vi "Main_04A.vi"() -> ()   [LabVIEW 2025]
uses:
  Utility/Universal Utility/TypeDefs_Utility/ENUM_8 Directions U-D-L-R.ctl
  Utility/Universal Utility/TypeDefs_Utility/Cluster_Row-Column.ctl
  b43e3300-6143-4e08-a70a-80936fe279ff.vi
  9e3f57c0-2ef8-4495-8287-c6a42a5fb955.vi
  <vilib>/Utility/error.llb/Trim Whitespace.vi
  <vilib>/Utility/error.llb/Trim Whitespace One-Sided.vi
  Utility/Universal Utility/TypeDefs_Utility/ENUM_4 Directions U-D-L-R.ctl
panel:
  out "Array":bool[][](array[boolean])
  out "MATCH":bool
  in  "Select Data":enum32{"Example", "Puzzle"}(tab)
  in  "EX Target":u32=13
  in  "Example":string="..@@.@@@@.\n@@@.@.@.@@\n@@@@@.@.@@\n@.@@@@..@.\n@@.@@@@.@@\n.@@@@@@@.@\n.@.@.@.@@@\n@.@@@.@@@@\n.@@@@@@@@.\n@.@.@@@.@."
  in  "Puzzle":string="@@..@.@.@..@@.@@@@@.@@@@@@..@@.@@.@@..@@@.@@@.@.@@@@.@@@.@@@.@..@.@@@@..@@@.@@..@@@.@@@..@@@@..@.@@.@@@.@..@.@@@.@@@..@@@.@.@@@@@.@.@.@@@@@@\n@.@@@@@@....@..@@@.@..@.@.@@.@@.@@..@@@..@.@@..@..@@@.@@@.@..@.@.@@..@@.@..@@.@@@..@.@@.@.@..@@...@@@@@@@@.@@@.@@@.@@.@@@@@@@..@..@@@.@.@@.@\n.@.@@@@.@@.@@.@.@.@@.@..@@.@@..@@@@@@@@@@@@...@@.@...@@@@.@.@@.@@@.@.@@..@@.@@.@@.@@..@...@@@@.@@@@@@@@@@@.@@@....@@@@@.@.@...@@.@@@@@@@.@@@\n@@@..@@@@.@@@@@@@@.@@@@@.@@.@....@.@..@.@@@@@@@...@@@@@@@@.@@...@.@@.@@@@@@.@....@@.@@@.@.@@..@@@.@.@@@..@.@.@@@.@.@@@@@@@@...@.@@@@@@.@..@@\n@.@@@@@.@@.@.@.@.@..@@@@.@..@...@.@@@.@.@@@@.@@.@@@@@@.@@@@@..@@..@.@.@@.@.....@@@.@@@.@..@@@.@@.@..@@@@.@.@@@@..@@@@@@.@@@.@@.@@..@@.@.@@@@\n@@.@@@@@.@@@.@@@@@.@@.@.@@@@.@@...@.@@@..@@.@@.@@@..@@@...@@.@@@@..@@@@@@@...@.@@@@@@....@..@@@@@.@...@.@.@@.@...@@@@.@.@@@.@@.@.@@@@.@.@@@@\n...@.@@.@@.@.@.@@@@...@@@@@@@@@.@.@@@.@@.@@@.@@.@@@@.@@@@@@@@@.@@..@..@.@@@@@@@@@@@@...@.@.@@@.@.@.@.@@@.@..@@@@@@@@@@@.@@.@...@@@@@@@@.@@@@\n..@@@.@.@.@@@@@...@@..@@..@@.@...@@@.@.@.@.@.@@.@.@@@.@@.@.@@@@.@.@@@@@@@.@@.@.@@@@@@.@.@@@@@@@@@@@.@.@@@@@.@@@@@@@@@.@...@@@.@@@@.@..@@@@..\n.@@@@.@@@.@.@@@.@@@..@@..@@@@@@.@..@.@@.@.@@@@@..@@@@@@@@.@.@@@.@@@@@.@.@@@@...@@.@@@.@.@@@@@@.@@.@.@@@@.@.@@@.@.@@@@@.@@@@...@@@@@@@@@@.@..\n@.@....@@.@..@@@.@.@..@@@@.@.@@.@..@@.@.......@.@@@@@@@.@@@@@@@@.@@@.@.@@.@@@@.@..@.@@@@@@.@@@@....@@.@@@@.@..@@@.@@.@.@@@@@@@@.@@@@.@.@@..@\n@@@@@.@@.@.@.@@.@..@@@.@.@@@@.@@@.@.@.@@@.@.@@@.@@@@@..@@@@@@..@@@@@@@@@@@@@@.@@@@.@@@@...@.@@@@..@@@@@@@.@@@@.@@.@@@@@@.@@@.@.....@@@@@@.@.\n@.@@...@@@.@@..@@@@..@@.@@.@...@@@@@...@@@@.@@@.@@.@..@@@@..@.@@@@..@@@.@..@@@@..@.@@.@.@.@@....@.@@..@@.@@..@@@@...@@.@..@@@@@@@...@@@..@.@\n...@.@...@@@..@..@.@@@@.@.@....@@@@@@.@..@@@@@.@@@@@@@@@@.@@@@@@@@.@@..@@@@@@@@@@@@@@.@.@...@@....@@.@@.@@@.@@@@@@.@.@..@@@@@@.@.@.@@..@@@@.\n@@@@.@@@@.@.@@.@.@..@@@..@@@.@@@@@..@@@@@@.@...@.@@@.@.@..@@@@@@.@@.@@@.@@..@@@@@@@..@@@@@@@@..@@..@@@@@..@.@.@@@.@@..@.@.@@@@@@@.@.@@@.@@@.\n@@@@@@@@.@@@@@@@.@@@.@.@.@@.@..@@@@@@@.@@..@@..@.@..@.@@@@@@..@.@.@@.@.@@@.@.@@@@..@@@@@@@@....@.@.@@@@@@@@@.@@@..@@@@@@..@@@@...@@@...@.@.@\n..@@@..@.@@.@.@@...@@@..@.@@@...@..@@.@@@@@..@@@@.@@@@.@@@.@@.@@.@@@@@@@..@.@..@.@.@@@..@@@@@...@@..@....@......@.@.@.@.@@@.@.@@@@@@@.@@.@@.\n.@@.@@@@@.@..@@@@@@.@....@@@.......@..@@@.@@@...@..@@..@@@@..@.@@@@.@@.@@..@@.@.@@@@.@@.@@.@@@@@...@@@@.@@@..@.@.@@@.@.@@.@@@..@@@..@@@@@..@\n@.@.@..@.@.@.@@.@@@@@@@@@@@@.@@@@.@@..@.@.@@@..@@@@.@@@@@...@.@@.@@@@@@@...@@..@@@@..@@....@.@@@.@.@@@@@.@@@@@@@..@@@@@@@@@.@@@@..@@@.@....@\n@@..@@.@@.@.@..@@...@.@.@.@@....@@@@@@.@.@@@@@@.@..@@@@@@.@@@@..@.@.@.@.@.@@.@@...@@@.@.@@.@@.@@@@@@@.@..@@.@.@.@@..@.@@@@@@@@.@@@@..@@...@.\n.@@..@@@@@@@.@.@@@@.@@@@@@@@.@.@@@@@@@@@.@@@@@.@@@@..@@@@..@.@@@@.@.....@.@@.@@.@@@@@..@@@@@.@@@@@.@@@.@@.@@@..@@@..@@@@.@@.@@@@@@@@@@@@.@@@\n.@..@@@@@@@@@@@.@@.@@.@..@..@@@...@@..@@@.@@.@.@@.@.@..@@.@@.@@@@@.@@@.@.@@@@.@@@@@.@...@@.@@.@.@@..@@@.@@@@@.@@@@@.@....@@@@@@@@.@@.@@@@@@@\n@..@@..@@@@.@@.@.@.@.@.@@@@..@@.@..@.@@@@@@@.@@..@@@@@.@@@.@@@.@.@@.@@.@@@.@@@@@@@@@@@@@.@@@@@@.@@@@@@@...@@@@@@@.@@@@.@.@.@@@.@@@.@..@@@..@\n@@@@@@@@.@.@@..@.....@.@@@...@.@@..@@@..@..@..@@@.@@@@@@@@.....@..@@.@.@.@.@@@@.@@.@@.@@@@@@.@.@.@@.@@@@@.@.@@@...@@.@@@@@@@...@.@@.@@@..@.@\n.@@@@@@..@.@@...@@@@@@@@@@@.@@@@@..@...@.@.....@@@.@.@@@.@@...@.@.@.@@@@@@.@@@@@@.@@@@@...@@@@.@..@@.@@@.@@.@.@@@..@@@@@@@@.@@@.@@..@.@.@.@@\n@.@@.@@@.@.@.@.@@@@@@@@.@@@@..@.@@@@@.@@.@@....@..@@.@..@@@....@@..@@.@@@@@@@@@....@@.@@@.@@..@...@@@@@@@.@@@@@.@@@.@@@@@@@@@@...@@.@.@@@@@@\n@@@@@@@@@...@.@.@@@.@@.@@.@.@..@..@..@..@.@.@@@.@@@@@@@@@...@@@@@@@@@@.@@@.@@.@@...@@@@@@@.@.@@.@@@@@.@.@@..@..@....@.@@@.@...@..@..@@.@@@@@\n@@@@@@@@...@@@.@@@....@@@.@..@@@@.@@@@@..@@@...@@.@.@@@.@@.@.@@.@.@@@@.@@.@@@@@@@@@@@@..@@....@@.@@@@@.@@@@@....@@@....@@@@@.@.@@.@@..@@@@@@\n.@@@@.@@@@....@..@.@@@@@.@@@@@@..@..@@.@@@@.@@@..@@@...@.@@@.@.@@@@@@@..@..@...@@@.@@@.@@@..@@@@@...@...@..@@@@@.@@..@@...@@@.@@@@@.@@@...@@\n@..@@@...@@@.@.@@@@.@@@@@@.@@@@.@@.@@@@@@@..@@@..@@@@.@@@@..@@@..@.@@@...@@.@@@@..@@@@@@@@.@@@.@@...@@...@.@..@.@.@@.@.@@@@.@@.@..@@..@..@@.\n@@@@@@@..@@..@@.....@@..@@@..@@@@@..@@@@@.@@@@@.@..@@@@..@.@@@@...@..@@@.@.@@@..@@@..@@@@@..@@@@.@.@.@@.@@@@@@...@@@@@@@@@@..@@.@.@@.....@@@\n.@@@@......@@@.@@..@@@.@..@.@@@@@@.@.@..@@.@@@.@@@@....@@@@.@@.@@@@@@@.@.@@@..@@@.@@@@@@..@@@.@@@@.@@@@@.@@@@@@@.@@.@@@@@@.@@@@@@@@@.@..@@@@\n....@@@@@.@.@@@@@@@@@.......@.@@@@@@..@@.@@@@.@@@..@@@.@..@@@.@.@@.@@@.@@..@@@.@@@@@@@.@.@@@@@@...@@.@..@.@@.@.@@.@@@@@.@@@@@.@..@...@@@.@@@\n@@@@@@@@@@@@.@@.@@@.@@.@@.@@@..@@@@@.@@@.@..@.@.@@.@@.@@@@@..@@.@@..@....@..@...@@@@@..@..@.@.@@..@...@@@@..@.@@@@@@@@.@@@@@@@@@.@..@.@@@@@.\n@.@..@@@@..@@.@@.@.@@@@@..@@@@@@@....@@.@@..@@.@@@@...@@@@.@@@@@@@@@@.@.@@.@..@.@@@@@@@@.@@@..@@..@..@@@..@@@@....@@@@@@.@@..@@@@@@@@@@@@@@.\n.@@.@.@.@@@@@@.@@@.@@@@.@..@.@@.@@@@..@@@@@@.@@@.....@.@.@....@.@@@@@.@@@@.@@@@@@@@@@.@@@.@@@@@@@..@@..@@.@...@.@@@.@.@.@@.@.@@@@@@..@@@@.@@\n@.@@.@@@@@@@@@.@.@@.@@@@@@@.@@....@@.@@.@@@@@.@@@@.@...@@.@@@@.@@@@@.@..@@@@@@@.@@..@@@@@..@@.@...@@.@@.@@@@.@@@@..@..@@@@@.@@@.@@.@@@@@...@\n@.@@@.@.@..@.@@.@.....@.@.@@@@@@@@@.@@@@@@@@@@.@..@.@@.@@...@@@.@.@@.@.@.@@.@@@..@@@@@@.@@@@@@@@@.@....@.@@@@@@.@@@@@.@@.@.@@@@@@@.@@@@@@@.@\n@.@...@@@...@@.@@..@@..@.@.@@..@.@.@..@..@@@@@@@..@@@@@@@@@@.@@.@@@.@@@@..@..@.@@..@@@.@.@.@@@.@.@.@@@@@@....@.@@@@@@@@@.@@@@@@..@@@.@@@.@@@\n.@@@@.@@@.@.@.@@..@@@.@@@@..@@@.@@.@@@..@@@.@@..@.@@@@@@..@@@@@.@@@.@@..@.@.@@@@...@@.@...@.@@@.@@@@.@@@.@..@@@@..@@@..@@.@@.@.@@.@.@.@@.@@@\n..@@@@..@@@..@.@@@@@.@..@.@@.@...@@@@@@@@..@.@@@@@@...@@@@.@.@@@....@...@@.@..@@@@@.@.@.@.@@.@@@@@.@@@@@..@@@@@@@..@@.@@.@@..@...@@@@@@@.@.@\n.@@@@.@@@@.@@@@@..@..@@..@.@.@@....@@@@.@...@@@@@@@@..@.@..@.@@@@@@@@@@@.@.@@..@.@@.@.@@@@@@.@@@.@@@.@@@..@@..@@..@.@@...@@.@..@..@.@@@.@.@@\n.@@@@@@@@@@@@.@@@.@@...@..@..@..@.@.@@@.@..@.@@...@@.@@..@@@@@@..@@@@@@@.@.@@@@@.@@.@...@@.@@.@@@@@@.@@@.@.@@@@..@...@@@@...@@.@@@@@@@@.@@.@\n.@@@@.@..@..@.@@@@@.@.@@@@.@.@.@.@..@.@@@@..@@@..@@..@..@@@@@.@.@@@@...@..@....@..@@.@...@@.@.@@@.@@@@.@@@.@@@@@....@@@@.@@@.@..@@@@@@@..@.@\n@@@@@@@@.@@@...@@..@.@.@.@@.@@.@@..@@@..@@.@@@@@@.@@.@@...@.@@@@..@@@@@..@@..@.@@@@@@@@@..@@...@@.@@@.@@@@@@@.@@..@@.@@@@.@...@.@.@..@@.@.@@\n@.@@@.@.@@@@@@@@@@@..@@...@.@@@..@@@@@..@.@@@..@.@@@@.@@@@@@@@@.@.@@@.@@@@@@@..@.@@...@@@..@@.@.@@.....@@@.@@.@..@@.@..@@@.@.@.@.@@@.@@.@@@@\n@.@.@....@@@.@@..@@@.@@@@@@@.@.@@.@.@@@@@@@.@@.@@@@@.@.@@....@.@@@..@@@@@.@@@@.@.@@@.....@@@@@@@@@@..@..@@@@@@..@.@@@@@@@.@.@@.@@@.@@@@.@.@@\n.@@@@.@@@.@..@@@.@@@.@..@@.@@.@.@@.@@@.@.@@@@@.@@.@..@.@.@@@@.@@@.@@.@@@..@.@.@@@..@@@@@@@@@@@.@@@@@@@@@.@@@@@@..@@@...@@@.@@.@.@@@@@@.@@@@@\n@@.@.@@@@@@@@@..@@...@@@@..@@@.@@.@.@.@@....@@..@@.@@..@@@.@@.@..@@.@@@@.@@@@@@@@.@@@@@@@@@..@.....@@@@....@@@@@...@...@..@@@@@.@@.@....@.@@\n.@@.@@...@@@@@@.@@.@@@@.@.@@@@.@@.@..@@@@.@...@@@@.@.@....@.@@@@@@@@@.@@..@@.@.@@@@@@.@.@@.@.@@@@@@....@.@@@@@.@.@.@.@@@@..@@@@.@.@..@..@@@@\n.@@@@@.@@@.@.@@...@@..@@@..@@...@@@@..@...@.@...@@.@.@@@@...@@@..@@@@@@@@@.@@.@..@.@.@@.@@@.@@@..@@@@...@@@@@@@..@.@@@@@@.@@.@.@@@@.@...@@.@\n@@..@.@.@@.@.@@.@.@@@..@@...@@@@@@@@@@.@.@@@@@@.@.@.@@..@@@..@...@@@@..@......@.@.@..@.@.@.@.@@@@.....@.@.@.@@.@@.@.@@@@@@.@@@@@..@.@.@..@@@\n.@@@@@@@@@@.@@@@..@.@.@.@@@@@@@@.@@@.@@.@@..@@..@@@.@@..@.@.@.@@@..@.@.@@@.@..@@@.@@.@.@..@@@...@.@@@@...@@@.@.@@.....@@...@.@@.@@@@@.@@@@@.\n.@@@..@@@@@@@.@@@.@@@@..@@@..@..@@@..@@@..@@.@@.@@@@@@@.@.@@@.@.....@@@@@.@@.@@..@@@@.@@....@@@..@@@@.@@@@@@.@@.@..@@@.@..@@..@..@@.@@@.@@..\n@@@@@@..@.@@@@@.@@@@.@..@.@@@@@..@@@@..@..@@@@@.@@@@@@@.@..@@..@@@@@@@@..@@@@.@.@@.@@...@.......@@.@..@@@@.@..@@@@...@.@@@.@......@@...@@@..\n@.@.@.@....@.@.@@.@@@@@@@.@..@.@..@@.@.@.@@@@@@..@...@...@.@.@.@.@@@@@@@@@..@@@.@@@@@@@@@.@..@@@@@@.@@.@@@@@@.@@.@@...@@@@@@.@@@.@@.@..@..@@\n.@@@.@@@@@@@@.@@@.@..@@.@..@..@@.@@@..@@@@@@.@@@@..@@....@@@@.@.@@.@@.@@@..@@@@@@@....@..@@.@@@@@..@..@...@@.@@@@@.@@.@@@@.@@@@@@.@..@.@@@.@\n@..@...@@@@..@@..@@..@@@.@.@@@@.@..@@@.@.@.@@@@@.@@...@..@@...@....@.@.@@@@@.@@@.@@..@@.@@@.@.@@..@@@@..@@@@@@@@@.@@@@@.@@.@@.@.@@.@.@.@@@.@\n@.@.@@@.@..@.@.@.@.@@@@@@@.@.@@.@..@@@.@@@@@@@...@@@.@@@.@@@@.@@@....@@@@@@@.@@.@.@@...@..@@.@..@.@@.@.@@@@..@@@.@@@@@@..@@@..@.@@@@@@@@@@.@\n.@@.@@@@..@..@@.@.@.@@.@@@@..@@.@....@@@@.@@@.@@@.@@@@@@@@.@@.@@@.@@@@.@@@@@@@@@.@@@@..@@.@..@@@.@.@@@@@@@@@@@.@@.@.@.@...@@@@@.@@.@...@@@@@\n.@..@@...@@.@@@@@@@@@@.@@@.@@.@@@@@@@.@@.@@@@.@@..@@.@.@@.@@@.@@@@.@.@@@@..@...@.@...@@@.@@@@@..@@@@@@@..@.@@@.@.@.@.@.@@.@@@@..@.@..@.@.@@.\n.@..@...@.@@.@..@@@@@@..@.@@@@@@...@@..@@.@@@@.@....@.@@@..@@@@..@@.@.@..@.@@.@.@.@@@.@..@.@@@@@@.@@@.@@.@.@..@@.@@.@.@@@.@.@.@.@@@.@@@.@@..\n.@@@.@.@..@..@@@..@@@.@@.@.@@@.@@@.@@@.@@@..@@@@@@..@@@@@@@.@@@@.@.@...@@@@@@@.@@@@...@..@@@@.@.@@@......@@@.......@@.@..@@@@@..@.@.@@@...@@\n.@@@@@@.@@@.@@@@@@@.@@.@@.@@@@@..@.@.@.@..@@.@.@.@@@.@.@@@.@@@.@@.@@..@@@..@@@@...@@..@.@.@@@..@@..@.@@@.@..@.@@@@@@@@@...@@@@.@@@@@@@.@.@.@\n@.@.@@.@@@....@@@@@@@.@@@...@@@..@.@@@@@@@@@@@@.@.@@@@@.@@@.@@.....@.@@@....@.@@....@@@@@@@.@@@@@.@@@.@.@.@@.@@@@@@@@..@.@.....@@@@@..@@@@.@\n@....@...@.@.@..@@@@@......@.@...@.@.@..@@.@@@@@@..@@@@.@.@.@.@.@.@...@@@@.@@@.@...@...@@@...@@@@@@@@@@@..@@@..@.@@@@@@.@@@@@....@@@.@@.@..@\n@@@@.@..@@@.@@@..@@.@@@@@@.@.@.@.@@@@@@@.@.@@.@@@.@@...@@.@.@.@@..@@@.@@@@@.@@.@.@@@@@.@@@@@@.@@.@@@@@.@.@@.@@....@@....@....@@@@.@@.@@@..@@\n@.@@@@@@@@@..@@@@@..@.@@.@..@@@.@@@@@@@@..@@@@@..@@@.@.....@@@..@.@@@@@@..@@..@@@.@.@..@.@@.@@@@@@.@.@@.@@@.@@.@@.@..@.@.@@@@..@.@@@@..@.@.@\n@@@@@.@.@.@@...@@...@@@@@@@@.@..@..@@@@..@@@..@.@@.@.@@@.@.@@@...@.@@@..@@@@@@@@@....@@@@@.@@@.@@..@@...@@@.@.....@@..@@@@@@@@@..@@@@@.@@@@@\n@@@..@@@.@@@@@@@@@@@@..@..@.@@.@@@@@@@@@@@@@.@@@@@@.@..@.@@@@@@@.@@@@@.@@@@@@@...@@@@@...@@.@.@@@@..@@@@@@.@@@@@..@@@@@@.@...@..@@@.@@.@.@@.\n.@@..@@@@@.@@.@@@@@@.@@@.@@.@.@@@@.@@..@@@....@@@@@@@.@@....@@@@@@.@@.@@...@..@@@@@@..@.@.@@@@@@@@@@.@@@@.@@@@.@.@@@@...@.@.@@.@.@@.@.@@@@..\n@.@@.@@.@@@@@@@@@.@@@@@@@.@@@..@..@.@...@..@..@.@....@@.@@.@@@@.@.@@.@@.@@.@.@@@@@@@@@@@.@.@@@..@@@..@@@.@@@@@@@@.@.@@@@@@@.@@.@..@@@@@@@@@@\n..@@..@.@@@@@.@@@.@@@.@.@@@@.@.@@@@@@@@@@@@@.@@@@...@@@@@@@@@@.@.@@.@...@@@@@..@@.@@@@..@@@...@..@@@.@@@.@@@..@@@@.@.@@.@@@.@.@.@.@@@.@@.@..\n@@..@@@@@...@@@.@@@@.@...@@@@@@@.@@@.@...@@@@@@@..@..@@@@@.@.@@.@.@@.@.@.@@@@@@...@.@....@@@..@.@@@@@@@@@@@@.@..@@@@@@@@@.@@.@@@@@..@@@@.@@.\n@.@@.@@..@...@@@@@@..@.@@...@@.@@@@@@.@.@...@@.@@@.@.@@@@@.@@@@@.@.@@@.@.@@@@@@@@@.@@@.@.@@@@@@@@@@@@.@.@@@.@@.....@.@@@@@@@@@@@@@@@..@...@@\n@.@.@.@.@.@@...@@@@@@.....@.@.@..@..@@@@@@@..@@@@@@....@@.@..@@..@.@@..@@@.@@.@@.@@@@@.@....@@@@....@.@@@...@..@...@@.@@@@@@@@@@.@@...@@@@.@\n@@@.@@@...@@@.@@@@@@@@.@.@@...@@@@..@..@@@@@..@@@@@@@@@....@@@@@.@@@....@.@.@.@.@@.@@@@..@@@.@@..@.@.@@@@@@@@@@@@@@@@.@.@.@@@@@....@..@@.@@@\n...@@@.@@.@@.@@.@@...@.@.@...@@.@@.@@.@..@@@@.@@.@@@@.@@.@@..@@@@...@@@@@.@..@.@@@@@@..@@..@@@.@.@.@@..@@@@@@..@@..@.@@@@@@@@.@...@@.@@.@@.@\n@@@@..@@.@@..@.@@@@@.@.@@@@.@@..@..@@.@.@@@@..@@@@@@@@@@@@@.@.@@@@.@.@@@@@@.@...@@@@.@.@@...@.@@@@.@@@..@@@..@.@@@@@..@.@@.@@.@@@@@@@@.@@@@.\n@@@..@@..@@@@@.@@.@..@@@.@..@.@@.@@..@.@.@@.@....@@@...@@@.@@@..@.@.@.@@@.@.@.@....@@....@@@@@.@@@@@@@.....@@..@.@@@.@@@@....@@..@@@.@@.@.@.\n@@.@..@@@@@@@.@.@@.@@@.@@@.@@.@@@@@@@@@@.@@@..@.@@@@..@@.@@.@.@.@@@.@.@@@@@@......@@@..@@@.@.@@.@@@@..@@.@@.@.@@..@.....@@@@@.@.@@.@.@.@.@.@\n@@@.@@@@..@.@@.@@@.@.@@@.@....@.@.@@..@..@@.@@@@@@.@@.@@@@.@@@@@@@@@@@@@..@.@.@@..@..@@.@@@@.@@.@@.@@..@@@@@@.@@@@@.@@.@@@.@@.@...@@.@@.@.@@\n@.@@@@@@@..@.@@@.@.@@@.@.@@@@@..@@@@@...@@@@.@@..@@.@.@...@@@@@@@@@@@.@@@@@@...@@@@@.@@@@@..@@@.@@.@..@.@@@@.@@.@@@.@@@.@@@.@.@@@@@@@@@..@@.\n@.@@.@..@@.@@@@@.@@.@@@.@..@..@@@.@.@.@@@@@.@@..@.@@....@@@@@.@..@@.@@.@@.@@.@@.@.@@.@@@.@@@.@@.@.@@@.@@@@@@@..@@@.@.@@.@.@@.@@@.@@...@.@@@@\n@@......@@@@@.@.@.@.@@@@..@@.@@@@@@@@@.@@@@.@@@.@@@.....@@@@@@@@..@@@@.@@...@@@@@@@@..@.....@.@@@..@.@@@@@@@@@.....@@@@@@@@.....@@.@@..@@.@.\n@@@...@@.@.@.@@.@@.@..@.@@.@@@@@..@..@.@@@@@@@.@@.@@@..@..@.@@@@.@@.@@@@@@@@@@@.@..@@@@.@..@@@@@.@.@@@@@@@@@..@@.@@@@...@@@@@@@.@@..@@.@@@@@\n.@.@@@.@@@@.@@.@@@@@...@@..@@@@@@@@@.@.@@..@.@@.@@@.@@@@@@.@@@@...@@.@@@..@...@@.@@@@.@....@@@.@....@....@@@@@@.@@@..@@.@@..@@...@@@..@.@@@.\n.@....@.@@@@@@@@@@...@@@@.@.@.@.@@@.@@@@@@@@@.@@.@@@..@.@.@@@@.@...@@@@..@.@@@@..@@.@@@@.@@@@@@.@@.@.@@.@..@@@@@@@@@@@@@@@@.@@@@@@.@.@.@.@..\n..@@@.@..@@..@@@@@@@..@@@.@@@@..@@..@@@@.@@@@..@@@.@@@.@@@@..@@..@.@.@.@@@@@@@...@@.@@@@@@.@@.@@@.@@@.@@@@@@@@.@.@@@@@@@@@.@.@....@@.@@@@@@.\n@.@@@.@@@@@.@@@@@.@@@...@.@@.@@@@@@.@..@.@@@@@@.@@.@@@@@@.@@@@@.@@@@@@...@@..@@@@@..@.@@@.@.@@.@.@.@@.@@@@.@.@..@@@.@.@@@...@@@..@@.@@@@@..@\n@@@.@@@.@@..@..@@@....@.@@@..@....@.@.@@@.@....@@@..@@.@@@@.@.@@...@..@.@@@.@@@@@@@@@..@.@@...@@@.@@@@@...@@....@@@@@@.@....@@@.@@.@@..@@@@@\n@.@..@...@@..@.@@@..@@@@@@.@..@@@..@@@@@.@@@@@@@.@..@@@@...@@.@@@@.@@@@@.@.....@@@@@.@@@@@.....@@.@..@@.@@@@@.@@.@@@@@.@@.@@.@@.@.@@..@.@.@.\n@..@@@@@@.@@...@.@..@@@@.@@@.@@@@@@@@.@..@@@@...@@@@@@@.@.@@.@@@@..@....@.@....@...@@.@@.@.@.@.@.@@.@@.@@.@@@..@@@@.@@@@.@@@.@.@@...@..@@...\n@@@@@@.@@@@@.....@@@@@@@@@@@..@.@@@@@@@@..@...@.@@.@@@@.@@@.@@@.@.....@.@@@.@@..@@@@...@@..@.@@@@.@@.@@@@..@@.@..@@@@@@@.....@@.@...@@..@.@.\n@@@.@@@@..@@.@.@@@@..@.@@.@@..@@@..@@.@@.@@...@@@@@..@..@@@@.@@.@@@@@.@@@..@@.@@@@..@.@.@...@@.@@@@@@..@@@@@@@..@@@@@@@.@.@.@.@.@...@@@.@@.@\n@@@@.@..@@.@.@.@@@.@..@@.@@@@@@@..@@@@@@@@@@@.@@@@@@.@@.@.@@.@@..@@@.@@@@@.@@.@..@@@.@@@@.@@@....@@@@@@@.@....@.@@@@@@@.@@@@.@@@...@.@@.@@@@\n@@.@.@@...@@@.@@..@@.@@@@.@@.@@.@..@.@..@@@@@@..@...@@..@@@.@.@@@@.@@.@@@.@.@@.@.@@@@@...@.@.@@@..@@@@.@@@@@.@...@@@.@@@@.@@.@...@.@@@.@@@.@\n@.@.@..@@@@..@@.@.@..@@@@@.@@@.@....@@.@..@@.@.@..@@..@....@@@.@@@..@@.@@@@@@.@.@.@@@@@.@@..@.@@.@@@..@@@.@@.@@@@..@@@@@@@@@.@@@@@@.@@@@.@.@\n.@.@@.@@@.@..@@..@@..@@@.@.@@.@@.@@.@....@@.@@.@.@@@@@.@@@.@.@....@.@@@.@@@@@@@@@@.@@@..@@@@....@@.@@...@.@@...@.@@....@...@.@@.@.@@..@.@@@@\n.@@@@@@.@@@@@@@..@@@@@@@@@@..@..@@@@@@@@@@....@.@@@@@@.@@@@@@@@@.@@..@.@...@......@.@@@@@.@.@.@@.@@....@@..@@@..@@.@@.@..@@@.@@...@@@@@@@@@.\n@@@.@@@@@@.@...@.@@...@..@@@@.@@@@@..@.@@.@@@@@@@....@@@.@.@@.@..@.@.@@.@.@@..@.@@@@.@....@...@@@.@@@@.@@@@@@@@.@...@@@@@@@@@@.@@@..@.@..@@@\n@@@@.@@..@..@@@@.@.@@@..@@.@@@.@@.@@.@@@..@@@@.@@@@@@.@@..@.@@@.@.@@...@..@@@...@.@@.@@.@.@@@@.@.@...@@@.@@@.@@.@.@@.@@.@@@@@@.@@@@.@@..@@@@\n.@.@.@@@@@@@@@.@...@..@@.@@@@@@@@@.@@@@.@@..@@.@@.@@@@.@@@@@@@..@@..@...@@.@@@@@@@@@.@@@@@@@@@@@@....@.@@@.@.@@@..@@..@@.@@.@@.@..@@.@.@@@@@\n.@@.@@@....@@...@@.@@@.@@...@@..@@.@@..@@@@...@@@@@..@@.@..@.@@@.@.@..@..@@@@.@@..@@......@.@@@@@@.@....@.@.....@@@.@@.@@@@..@@.@@@@..@@..@@\n..@.@@@@@.@@.@..@..@@.@@@@.@@@...@..@@@.@..@@@.@@@.@@...@@@@@@.@@.@.@@@@..@@@@@.@@@.@.@@@@@...@...@@@@.@@@@@.@@@@@@.@@@.@@@@@@..@....@.@....\n......@.@@@@@@@..@@@..@@@@@.@@@.@@@.@@.@.@.@@..@@@@.@.@@...@.@@@@.@@.@.@.@@@@@.@@@@@@@...@@.@@@@@..@@@.@@@.@.@@@@...@@@@@@.@@@.@@@@.@..@@@.@\n@.@@@@.@@.@@.@.@@.@@@@@@@@@@@@@@@@@@@@@@.@@@@.@.@.@@@@.@..@@@..@.@..@@@@@..@@@@@.@..@@.@@@@@@.@@@@@@.@@.@@@@@.@@@.@@@@.@.@@@@@@..@@.@@..@@@@\n.@@@@.@@@@@@@@.@@@@@.@..@.@..@..@@.@@@@@...@@@.@@@@@@.@@@@@@@@.@.@@@@..@@..@@@.@@@@@@.@.@@@@@@@.@@@.@..@.@@.@.@..@@@.@@@@@.@@@@@...@@@.@@.@.\n@...@@@@..@@.@@@.@@@.@@@@@.@@@....@@@@@@@@@@.@@..@.@.@.@.@@..@.@@@@@.@@.@.@@@@@.@@@.......@..@@......@@..@@.@@@.@@@@@@.@.@@@@@.@@@@.@@@@..@.\n.@@....@..@.@.@@@@@@@@@@@@..@@@@.@@@@@@@@@..@@.@.@@@@.@@.@@@@@@@.@@@..@.@.@@@@.@.@@@@@@@@.@@@@..@@@..@@@.@@@.@@@@......@@.@@..@@.@@@@.@...@.\n@@@@@@@@@@@@@@@@@@.@@.@...@@.@..@@.....@@@@@@..@@.@.@@..@..@@@...@@....@@@@@.@@@@.@@.@@@@.@..@@.@@.@@@.@@@......@...@...@@@@@@@@@@@.@@@@@.@@\n@@...@@@.@@.@.@.....@.@@@@@@@.@.@.@@@..@@@@@..@@.@@@@@@@@@@@@@@@.@@..@@@@...@@@.@@.@@.@@@@@.@..@@@.@@@@@..@@....@.....@@@..@@@@@@@@....@@@.@\n@@@@.@.@@@@@@@@..@..@.@@@@.@.@@..@@@@@@@.@@@@.@..@@@@@.@.@.@@@@@@..@.@.@...@@@@@@@@....@.......@...@@@@@@@.@.@..@@@@@..@@@@@@.@@@@@@.@@.@@@@\n@.@@@@@.@@@@..@..@.@@..@@..@@@..@@.@@...@@@.@.@@.@@@@@@@@@@..@@.@@@@@@.@@@..@@.@@@@@@@.@.@@..@.@..@@.@@@@.@@.@@@..@@.@@@.@..@@@@.@@@@.@.@@@@\n.@@@@@@@....@...@.@.@@...@@@@....@..@.@@@@.@.@@@@@.@@.@.@@@....@@.@@.@.@...@@.@...@.@....@@@.@@.@@@@.@@@.@.@.@.@@.@@.@@@@.@@@@@@.@@@@.@@@@@.\n@@@.@@@@.....@.@.@@@.@@....@@..@@.@@@@.@@.@@.@.@@.@@@@@@@@@@@@@@@..@..@@@@@@..@@@.@@.@..@...@@@.@@@@.@@@.@...@@@@@@@.@@@.@@.@@.@.@@@@@@@@.@@\n..@@@.@.@@.@@.@@.@@.@@...@@.@@..@.@.@.@..@@@@.@@..@@@@@@@@.@@@@@@@@.@.@.@@.@.@@..@@.@@@@@.@@@...@@@.@.@..@..@@@@@.@@..@@@@@@...@.@...@@@@@@.\n@@.@.@@..@@@@@@@.@.@@@@.@.@.@.@@@.@.@@@..@.@.@.@@.@@@@@@@@..@.@@.@....@.@@@@@@@@@@..@..@@@@@@@..@.@@@.@@@@@@@.@@..@.@@@@@@...@@@...@@@@@...@\n@@@@@...@@@@..@@@@@@@@@@.@@@.@@@@@@.@.@@.@@...@..@.@@@...@@@..@@.@.@@@@@@@@@@...@@.@@.@@@.@@@.....@@@@@.@@@@@@@@.@@@...@@.@@..@.@@@@@@@.@@@@\n...@@@@@.@.@.@.@..@@@@.@@@@@@@@@@...@.@.@@@...@@@..@@@@@.@@@@@@@@@@@@@.@@@@@@.@...@@@@.@@@@@.@.@@.@...@@.@@.@@@@@@@@@@@@@.@@..@.@@@@.@@@.@@@\n@@.@@..@@@@.@@..@@@.@@.@.@@@@.@@@.@@@..@@....@@@@..@@@...@@@.@@@.@.@@@.@@..@@@@@..@..@@..@@..@.@..@..@.@@@@.@.@.@@@@@@@.@@.@@@@@@..@@..@.@..\n@@@.@@.@@@.@@@.@..@.@@...@@.@@@.@..@.@@.@....@@@.@.@@@.@.@@.@@.@@.@@.@.@.@@.@..@.@.@@.@@.@@.@.@@@@@...@@@@..@@.@@..@.@@@@@@..@@@@.@@@@..@@..\n@@.@.@@@@@@@@@@..@@..@..@@@@@..@@@.@.@@@.@@@@.@@....@@.@.@@..@@.@@@@.@@.@@@@.@@.@@.@@@@.@...@@.@..@@@..@.@.@@.@@@@.@.@@@@.@.@@.@.@..@.@@.@.@\n@@@@@..@@.@...@@@@@.@@@.@@@@@@@.@@@.@@@@@@@@@@@.@@.....@..@..@.@@@@@@@@@.@@@.@@.@@..@.@........@..@.@@@@@@@@.@@.@.@.@@.@@@@.@....@@.@.@@@@.@\n@@@.@..@.@@.@@@@@..@@@@.@@..@@@@@@@@@@@.@@@@@@@..@@.@@.@@@@@@@@.@@@@@...@.@..@.@..@..@@@.@@.@@@.@@.@@.@....@@@@@@@@@.@@..@.@@@@...@.@@.@@@@.\n.@.@@...@@.@@.@.@@@@.@@..@@..@..@@.@@@.@@@@.@.@@.@.@@@@@@@..@@@.@@@@@@@@.@@.@@@..@..@@@@@.@@@.@.@@@@.@...@@@@@@@@@@.@@.@@.@@@.@@@@.@.@@..@..\n@..@.@..@@...@.@@@@..@@.@@@.@@@@@.@.@@@@..@@@@@.@@@@.@.@@.@@.@@@@.@@@..@@@@@..@..@@@@@@@.@...@@@@..@@@@@@@.@.@...@.....@@@@@..@.@.@@.@@@@@..\n.@.@@@@...@@@.@@@@@.@@@@@@.@@@@@@..@@..@@@@.@@@@@@@@@@@@@.@@@@@@..@@@@@.@@@@@@@@@.@...@@@@@@@.@.@@.@.@@@..@@@@@@@..@..@@@@@@@@..@@@...@@@.@.\n.@@@@..@@@@@@@@@@@@@@...@.......@.@.@@@@@@.@.@@@@@@@@@@@...@.@@@@@@.@.@@@@@.@.@@@@@.@.@@..@..@.@@@.@@..@@@@..@@@@@@.@@@@.@@@@..@@@.@..@..@@@\n...@@@.@..@@@@@.@@@@@@@.@.@.@....@@@@.@@@.@@@.@@@@@.@.@@@.@@@@@@@@.@@@@..@@.@@...@@@@@@@@@@@@@@@@.@@@@.@@@..@@@@.@@.@..@@...@@@.@@@@.@..@..@\n@..@.@@@@@@@..@@@@..@@@@..@.@@@@@@@@@@@.@@@@@@@@@@@@....@@.@@@@@@@@@@@@@@@@@.@@.@.@.@@.@.@.@@@@@@@@@@@@@@@...@@@@@.@@...@@@...@@..@@@@..@.@@\n@.@....@@@@@@@@@@@.@@@.@@.@@@@.@..@@@@@@.@@..@@@@@@...@.....@.@@...@@..@@...@@@@@@@@@@.@@@@@..@...@.@@.@@@.@@@@...@@@@@..@@@@..@@@@@.@@@@...\n@@..@@@@@@@@@@.@.@@@....@@@@@@.@@.@@@@@..@@@.@@..@.@.@@@@@@.@@@@@@.@@...@@@@@@@@@.@@@@@..@@@.@@@.@.@@@@@@@@@@.@..@.@@@@.@@@..@@@@.@@@..@..@@\n@@@....@..@@@@@@@@@@.@...@@.@@@@@@@@@@@@@..@@..@@..@@@..@.@@.@@@@.@@.@@@@.@@.@.@@@.@..@@@@@@@@.@.@@@.@@@@@@@@.@@.@@@.@@@.@.@.@@@@..@@@.@@.@.\n@@@@.@@@..@@@@@@@...@@@@@.@@@.@@@@@@@@@.@@.@.@@@.@@@.@.@.@@@@.@@@@@@.@@.@@....@@@@@@@@@.@@@.@@@.@@@..@@....@@@@.@.....@@@..@@@@@..@.@@.@@@@.\n@@.@@@@.@.@@.@@.@@@@@@@@@@@.@.@@.@.@@.@@@@...@@.@.@@@@@@.@.@@@@@@@..@.@@.@@@@...@@..@@@@@@@@@.@@@.@@.@@.@.@..@.@@@..@@.@@@.@...@.@@.@@..@@@.\n@@.@@@@@@@@@@@.@@@@.....@.@@@@.@@.@@@@@.@@@@...@@@.@.@@@@@@@@@..@@.@.@.....@@@@@@@@@@@@@@@@@..@.@@@.@@@@@.@@@.@.@@@@@.@.@.@@@@@@.@@@.@..@@.@\n@.@.@@@@@.@.@@...@@@@@@..@@.@@@@@@.@@..@@@@...@...@.@.@@@@@@@@@@@@@@...@@@..@.@@.@@.@.@@.@@...@@@@@..@@@...@.@@.@@@...@@@@.@@.@.@@..@.@@@@@.\n@@@.@@.@@@@..@@@@@@.@@....@.@.....@@.@.@@.@@.@@@@@...@..@@...@@.@@@@@.@...@@@@.@@.@..@@.@.....@@@@@@@@@.@.@@@...@.@.@.@.@@@...@@@@@@..@@@@@@\n@.@.@@@@@@@@@@.@.@@@..@..@.@.@..@.@@@@.@@@@@@.@@@@@@...@.@.@@@.@.@@@.@.@@..@@.@@@.@.@.@@.@..@@.@..@@@@@..@@..@@.@@@..@..@@@...@@@@.@..@..@@.\n.@@@@@@@..@@@.@@.@.@@@@.@.@@@@..@@..@@@..@.@@@.@@@@@@@.@@..@..@..@@@..@@@.@@@@.@@@.@@..@@@.@.@@@@.@@@@@...@.@@.@@.@@@@..@..@.@@...@.@@..@@.."
  in  "Puzzle Target":u32=1547
  out "Answer":u32
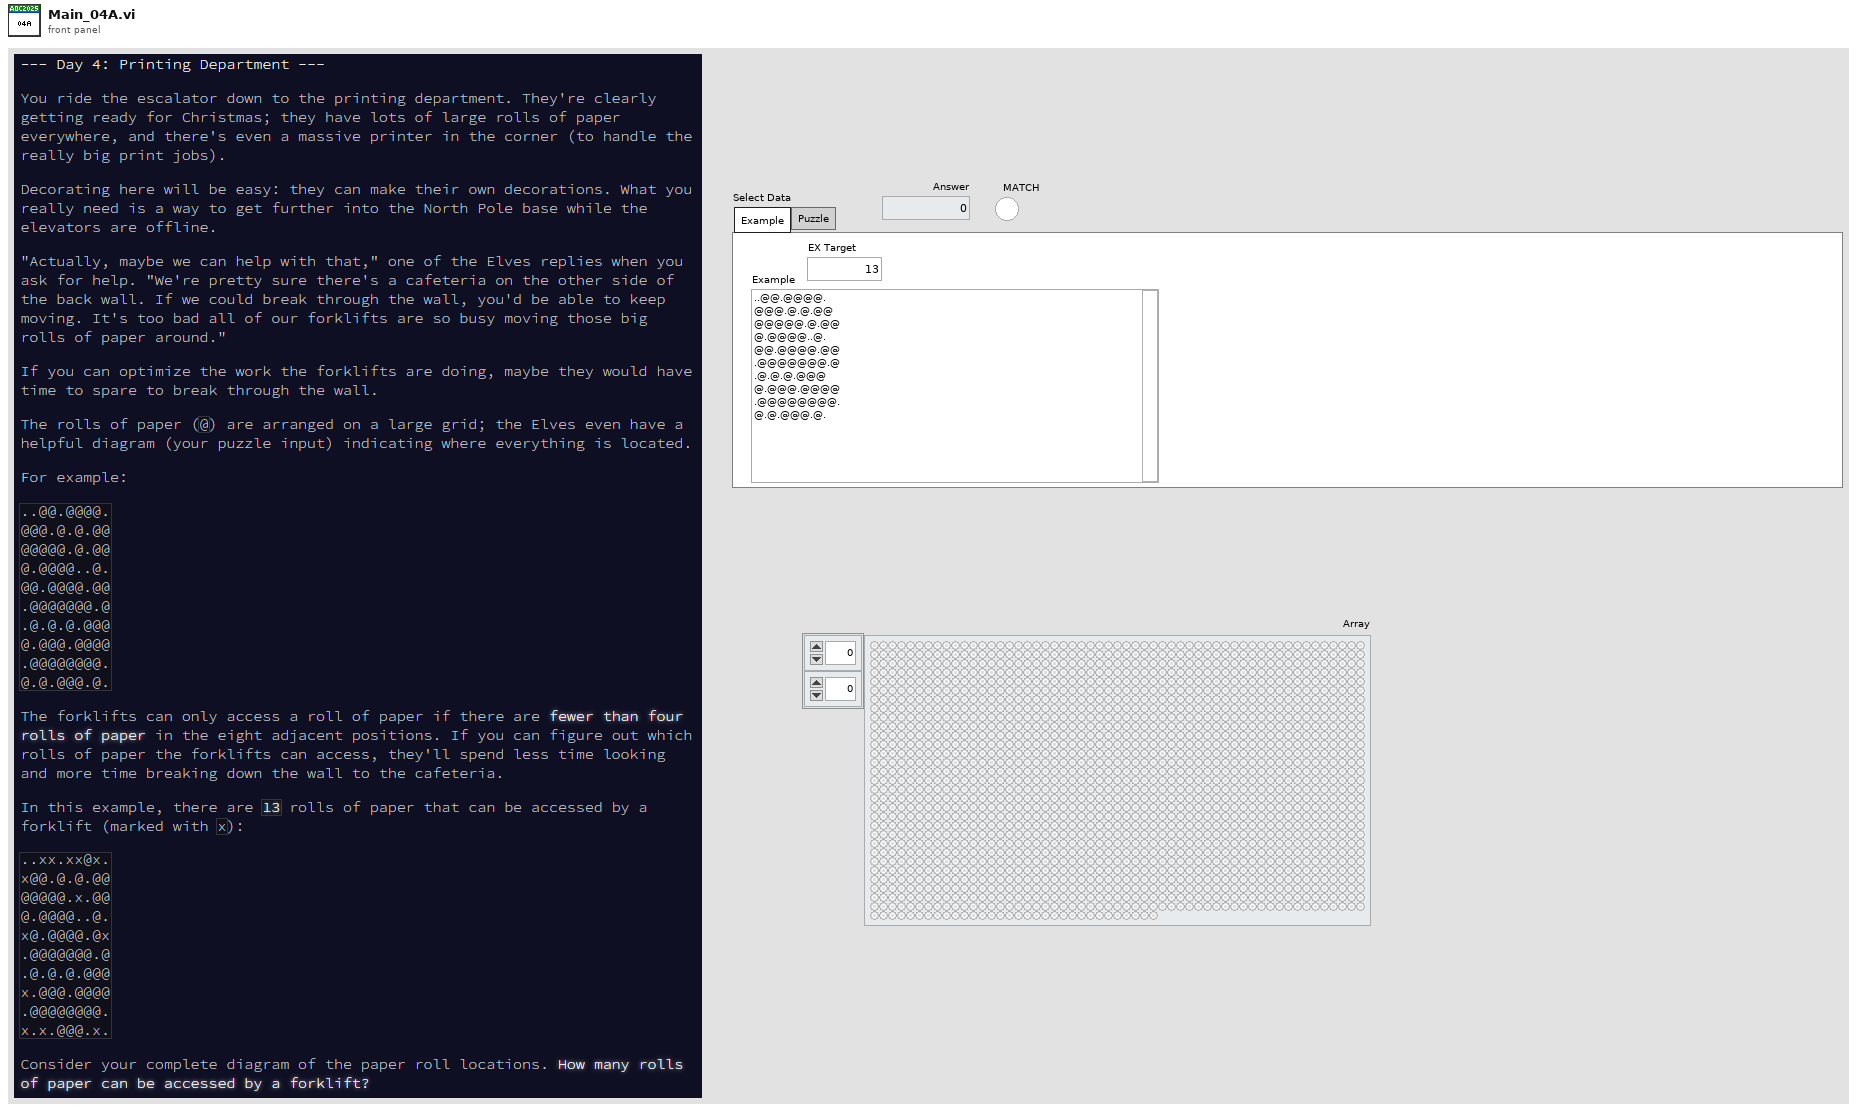
[diagram p1: front panel]
types:
  T1 = typedef "ENUM_4 Directions U-D-L-R.ctl" = enum16{"Up;-1,0", "Right;0,1", "Down;1,0", "Left;0,-1"}
  T2 = typedef "Cluster_Row-Column.ctl" = cluster{"R":i32, "C":i32}
  T3 = typedef "ENUM_8 Directions U-D-L-R.ctl" = enum16{"Up;-1,0", "Up-Right;-1,1", "Right;0,1", "Down-Right;1,1", "Down;1,0", "Down-Left;1,-1", "Left;0,-1", "Up-Left;-1,-1"}
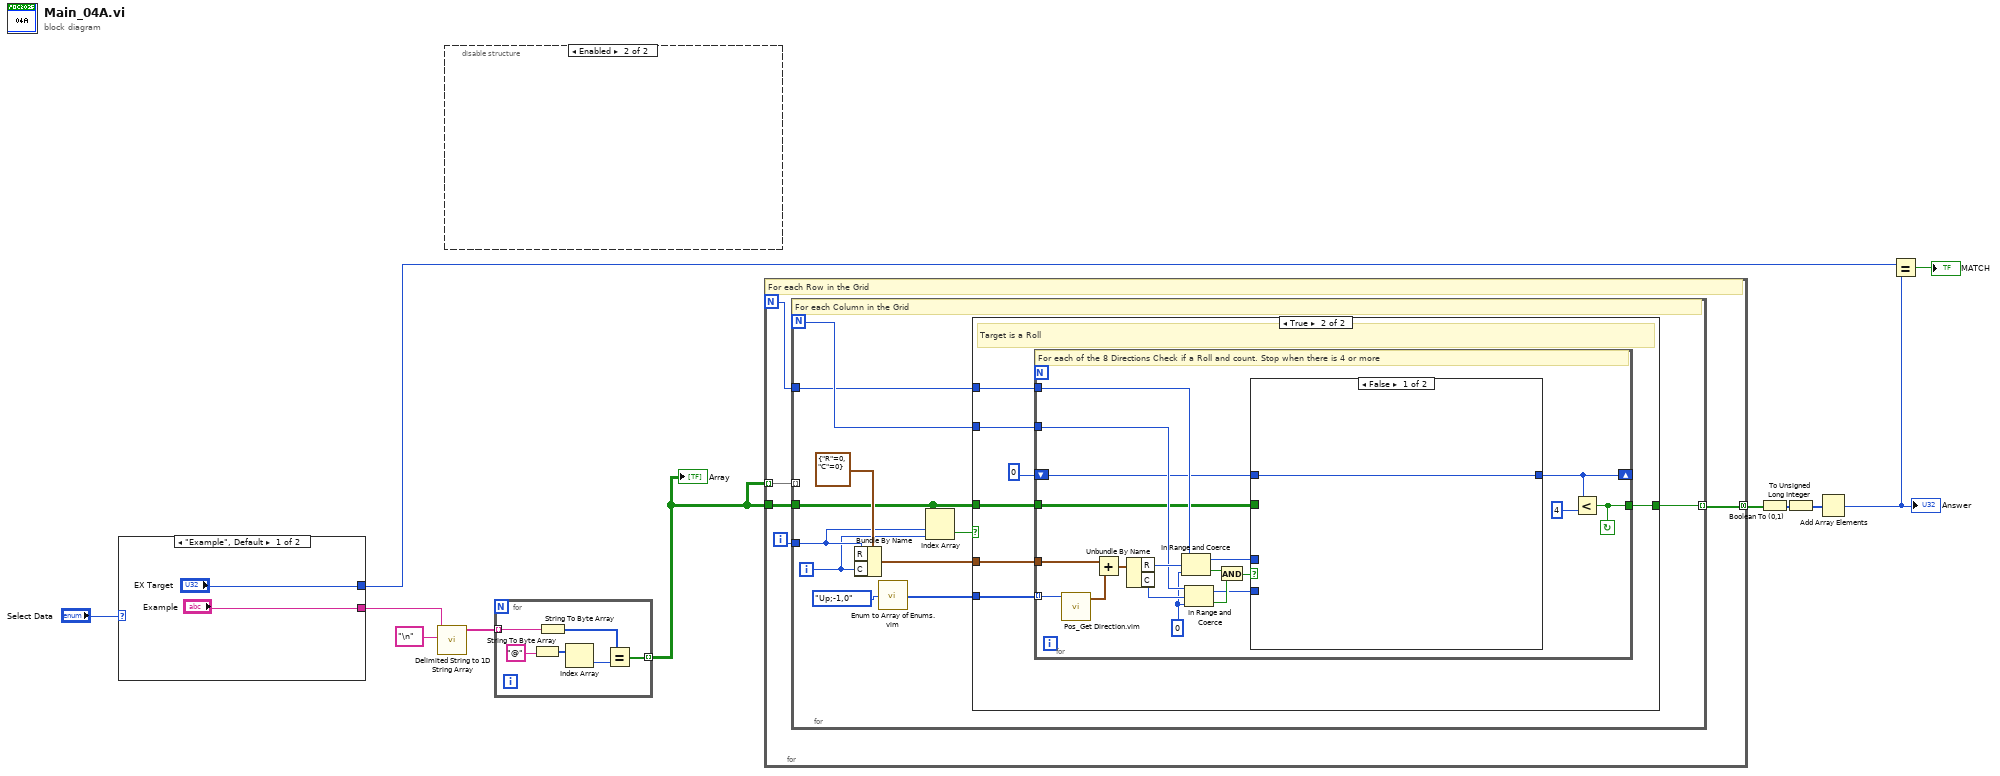
[diagram p0: block diagram]
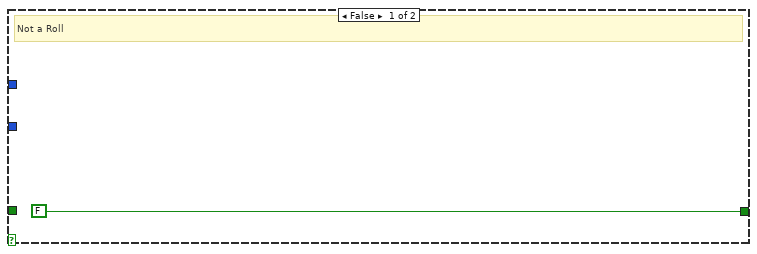
[diagram p2: hidden frame]
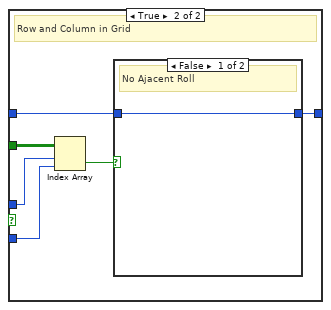
[diagram p3: hidden frame]
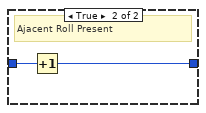
[diagram p4: hidden frame]
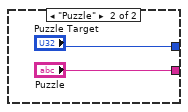
[diagram p5: hidden frame]
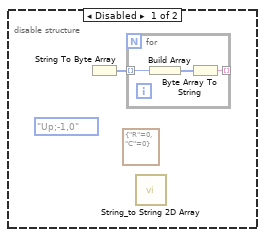
[diagram p6: hidden frame]
diagram:
  n1 = case shown="\"Example\", Default" "Select Data" {
    tunnel: ["Example" "Puzzle"] -> w9
    tunnel: ["EX Target" "Puzzle Target"] -> w6
    frame "Example", Default {
    }
    frame "Puzzle" {
    }
  }
  n2 = call <vilib>:"Delimited String to 1D String Array.vi"("delimiter"="\n" ("delimiter (Tab)"), "delimited string"=w9) -> ("string array"=w10:string[])  [unwired: 9 in]
  n3 = disable-structure shown="Enabled" {
    frame Disabled {
      (unwired) ENUM_4_Directions_U-D-L-R."Up;-1,0" ("Direction")
      (unwired) T2 {"R"=0, "C"=0} ("Position")
      n4 = String To Byte Array() -> (unsigned byte array=w16:u8[])  [unwired: 1 in]
      n5 = for {
        tunnel: w16 -> [w19] mode=indexing
        tunnel: [w17] -> _ mode=indexing
        n6 = Build Array(w19) -> (w18:u8[])
        n7 = Byte Array To String(unsigned byte array=w18) -> (string=w17:string)
      }
      n8 = call "String_to String 2D Array.vi"() -> ()  [unwired: 11 in, 1 out]
    }
    frame Enabled {
    }
  }
  n9 = for {
    tunnel: w10 -> [w21] mode=indexing
    tunnel: [w20] -> w1 mode=indexing
    n10 = String To Byte Array(string="@") -> (unsigned byte array=w23:u8[])
    n11 = String To Byte Array(string=w21) -> (unsigned byte array=w25:u8[])
    n12 = Index Array(array=w23) -> (element=w24:u8)  [unwired: 1 in]
    n13 = Equal?(x=w25, y=w24) -> (x = y?=w20:bool[])
  }
  "Array" <- w1
  n14 = for {
    N -> [w28]
    tunnel: w1 -> [w30]
    tunnel: [w27] -> w5 mode=concatenating
    tunnel: w1 -> [w26] mode=indexing
    i -> [w29]
    # "For each Row in the Grid"
    n15 = for {
      N -> [w37]
      tunnel: w30 -> [w34]
      tunnel: w29 -> [w33]
      tunnel: w28 -> [w36]
      tunnel: [w35] -> w27 mode=indexing
      tunnel: w26 -> [_] mode=indexing
      i -> [w32]
      # "For each Column in the Grid"
      n16 = Bundle By Name(cluster=T2 {"R"=0, "C"=0} ("Position"), "R"=w33, "C"=w32) -> (w38:T2)
      n17 = call "Enum to Array of Enums.vim"("enum"=ENUM_8_Directions_U-D-L-R."Up;-1,0" ("Direction 8")) -> ("array of enums"=w40:T3[])
      n18 = Index Array(array=w34, index (row)=w33, index (col)=w32) -> (element=w31:bool)
      n19 = case shown="True" w31 {
        tunnel: w40 -> [_ w49]
        tunnel: w38 -> [_ w48]
        tunnel: w37 -> [_ w46]
        tunnel: w36 -> [_ w45]
        tunnel: [FALSE w44] -> w35
        tunnel: w34 -> [_ w43]
        frame False {
          # "Not a Roll"
        }
        frame True {
          # "Target is a Roll"
          n20 = for {
            tunnel: w49 -> [w68] mode=indexing
            tunnel: w48 -> [w67]
            tunnel: w43 -> [w54]
            shift-right: [w52] -> _
            shift-left: 0 -> [w53]
            tunnel: w46 -> [w62]
            tunnel: w45 -> [w61]
            tunnel: [w50] -> w44
            stop <- w50 continue-if-true
            w60 = 0 ("lower limit")
            # "For each of the 8 Directions Check if a Roll and count. Stop when there is 4 or more"
            n21 = call "Pos_Get Direction.vim"("Direction"=w68) -> ("Position"=w66:T2)  [unwired: 10 in]
            n22 = Add(x=w67, y=w66) -> (x+y=w65:T2)
            n23 = Unbundle By Name(w65) -> ("R"=w64:i32, "C"=w63:i32)
            n24 = In Range and Coerce(upper limit=w61, x=w64, lower limit=w60) -> (coerced(x)=w55:i32, In Range?=w59:bool)
            n25 = In Range and Coerce(upper limit=w62, x=w63, lower limit=w60) -> (coerced(x)=w56:i32, In Range?=w58:bool)
            n26 = And(x=w59, y=w58) -> (x .and. y?=w57:bool)
            n27 = case shown="False" w57 {
              tunnel: w56 -> [_ w73]
              tunnel: w55 -> [_ w74]
              tunnel: w54 -> [_ w75]
              tunnel: w53 -> [w69 w71]
              tunnel: [w69 w70] -> w52
              frame False {
              }
              frame True {
                # "Row and Column in Grid"
                n28 = Index Array(array=w75, index (row)=w74, index (col)=w73) -> (element=w72:bool)
                n29 = case shown="False" w72 {
                  tunnel: w71 -> [w76 w78]
                  tunnel: [w76 w77] -> w70
                  frame False {
                    # "No Ajacent Roll"
                  }
                  frame True {
                    # "Ajacent Roll Present"
                    n30 = Increment(x=w78) -> (x+1=w77:i32)
                  }
                }
              }
            }
            n31 = Less?(x=w52, y=4) -> (x < y?=w50:bool)
          }
        }
      }
    }
  }
  n32 = Boolean To (0,1)(Boolean=w5) -> (0, 1=w4:i16[])
  n33 = To Unsigned Long Integer(number=w4) -> (unsigned 32bit integer=w3:u32[])
  n34 = Add Array Elements(numeric array=w3) -> (sum=w2:u32)
  "Answer" <- w2
  n35 = Equal?(x=w6, y=w2) -> (x = y?=→"MATCH":bool)
